vi "Set ICreate Action Point.vi"(8 "Error In":errorcluster, 10 "ICreate Action Point":refnum<class "ICreate Action Point.lvclass">) -> (0 "Error Out":errorcluster)   [LabVIEW 2019, in "Instrument Manager.lvclass"]
uses:
  Instrument Manager.lvclass
  Instrument Manager.lvclass/Instrument Manager.ctl
  Interfaces/ICreate Action Point/ICreate Action Point.lvclass
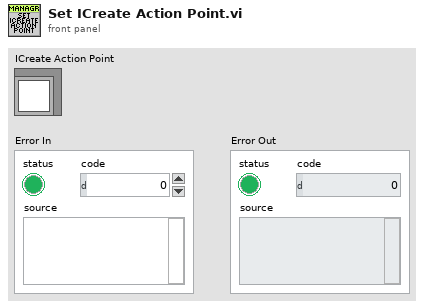
[diagram p1: front panel]
types:
  T1 = typedef "Instrument Manager.lvclass/ObjectAttributes.ctl" = cluster{"ICreate Action Point":refnum<class "ICreate Action Point.lvclass">, "IInstruments":map{string, refnum<class "IInstrument.lvclass">}, "IVirtual Instruments":map{string, refnum<class "IVirtual Instrument.lvclass">}, "Instrument Configurations":map{string, refnum<class "Config from JSON.lvclass">}, "Virtual Instrument Configurations":map{string, refnum<class "Config from JSON.lvclass">}, "Action Point Configurations":map{string, refnum<class "Config from JSON.lvclass">}, "Action Points":map{string, refnum<class "Action Point.lvclass">}}
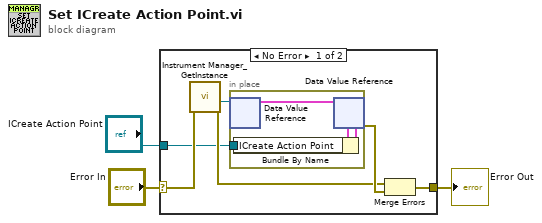
[diagram p0: block diagram]
diagram:
  n1 = case shown="No Error" "Error In" {
    selector: "Error In" -> [w9 w13]
    tunnel: [w6 w13] -> w2
    tunnel: "ICreate Action Point" -> [w4 _]
    frame No Error {
      n2 = call "Instrument Manager_GetInstance.vi"("Error In"=w9) -> ("Error Out"=w7:errorcluster, "DVRRefOut"=w5:refnum<data-value>)  [unwired: 6 in, 3 out]
      n3 = in-place {
        in-place-border: w4 -> [w12]
        n4 = in-place-dvr #1(w5) -> (w11:T1)  [unwired: 1 out]
        n5 = Bundle By Name(cluster=w11, "ICreate Action Point"=w12) -> (w10:T1)
        n6 = in-place-dvr #1(w10) -> (w8:errorcluster)  [unwired: 1 out]
      }
      n7 = Merge Errors(w7, w8) -> (w6:errorcluster)
    }
    frame Error {
    }
  }
  "Error Out" <- w2
